vi "3-2 생산자소비자(이벤트).vi"() -> ()   [LabVIEW 2014]
uses:
  <vilib>/Analysis/NI_AALBase.lvlib
panel:
  in  "기다림":i32
  out "웨이브폼 그래프":dbl[](graph)
  in  "정지":bool
  in  "확인 버튼":bool
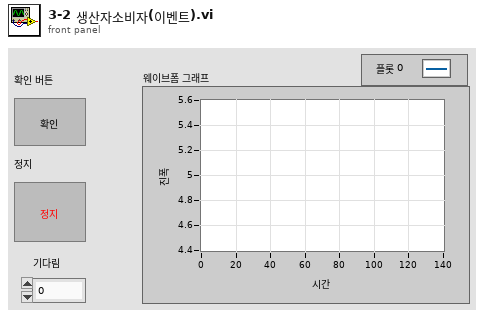
[diagram p1: front panel]
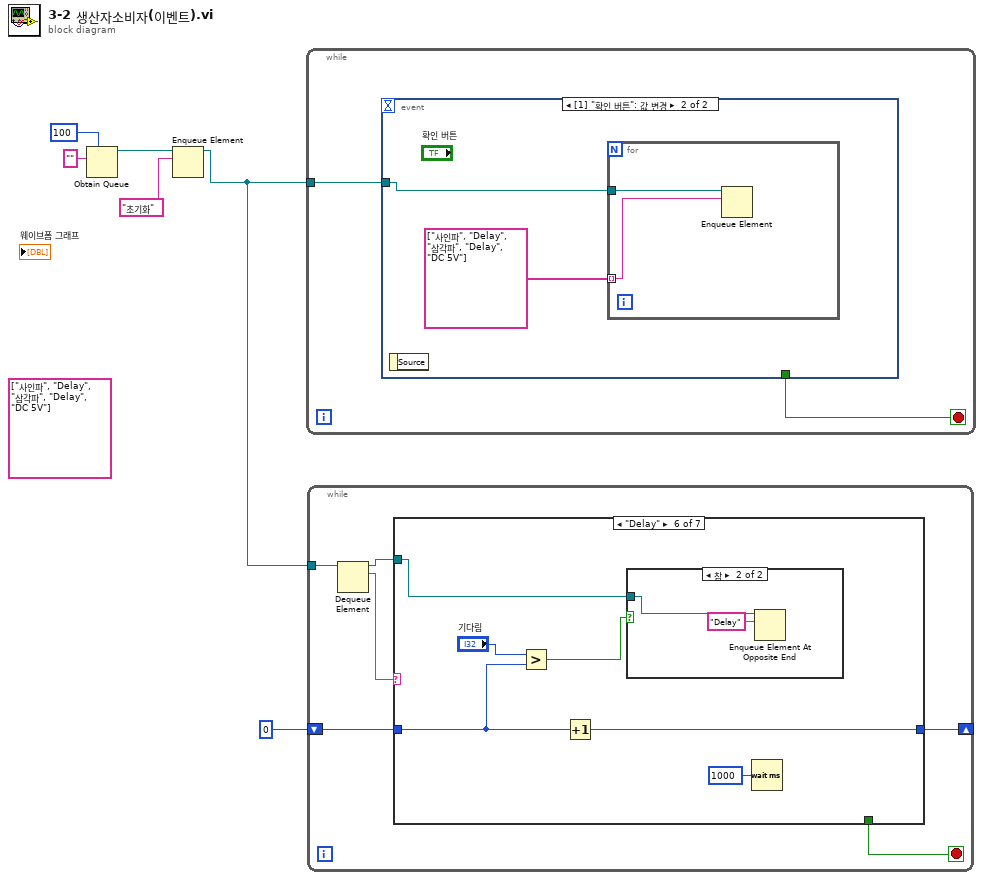
[diagram p0: block diagram]
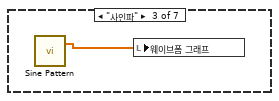
[diagram p4: hidden frame]
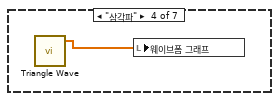
[diagram p5: hidden frame]
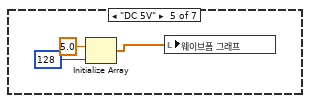
[diagram p6: hidden frame]
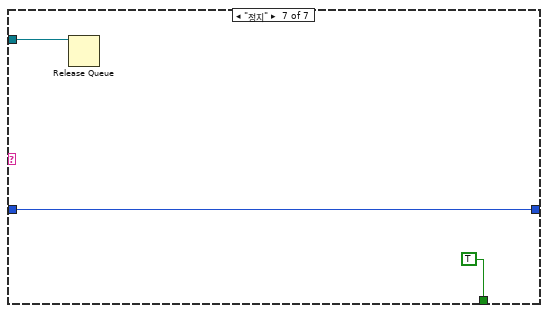
[diagram p8: hidden frame]
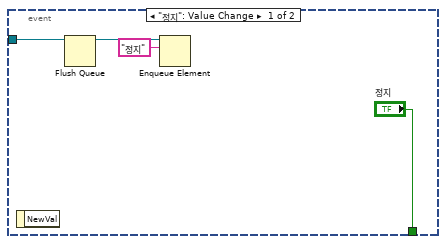
[diagram p9: hidden frame]
diagram:
  (unwired) string[] ["사인파", "Delay", "삼각파", "Delay", "DC 5V"]
  n1 = Obtain Queue(max queue size (-1, unlimited)=100 ("최대 큐 크기(-1,제한없음)"), element data type="" ("원소 데이터 타입")) -> (queue out=w4:refnum<queue>)  [unwired: 3 in, 2 out]
  n2 = Enqueue Element(queue=w4, element="초기화" ("원소")) -> (queue out=w3:refnum<queue>)  [unwired: 2 in, 2 out]
  n3 = while {
    tunnel: w3 -> [w7]
    stop <- w8 stop-if-true
    n4 = event shown="[1] \"확인 버튼\": 값 변경" {
      selector: _ -> [_ _]
      dyn-events: _ -> [_ _]
      timeout: _ -> [_ _]
      tunnel: ["정지" _] -> w8
      tunnel: w7 -> [w9 w14]
      event "정지": Value Change {
        n5 = event-data() -> ()  [unwired: 1 in, 1 out]
        n6 = Flush Queue(queue=w9) -> (queue out=w11:refnum<queue>)  [unwired: 1 in, 2 out]
        n7 = Enqueue Element(queue=w11, element="정지" ("원소")) -> ()  [unwired: 2 in, 3 out]
      }
      event "확인 버튼": Value Change {
        n8 = event-data() -> ()  [unwired: 1 in, 1 out]
        n9 = for {
          tunnel: w14 -> [w16]
          tunnel: string[] ["사인파", "Delay", "삼각파", "Delay", "DC 5V"] -> [w15] mode=indexing
          n10 = Enqueue Element(queue=w16, element=w15) -> ()  [unwired: 2 in, 3 out]
        }
      }
    }
  }
  n11 = while {
    tunnel: w3 -> [w22]
    shift-right: [w17] -> _
    shift-left: 0 -> [w18]
    stop <- w19 stop-if-true
    n12 = Dequeue Element(queue=w22) -> (queue out=w20:refnum<queue>, element=w21:string)  [unwired: 2 in, 2 out]
    n13 = case shown="\"Delay\"" w21 {
      tunnel: w20 -> [_ _ _ _ _ w33 w38]
      tunnel: [_ _ _ _ _ _ TRUE] -> w19
      tunnel: w18 -> [_ _ _ _ _ w30 w36]
      tunnel: [_ _ _ _ _ w32 w36] -> w17
      frame "기본", Default {
      }
      frame "초기화" {
      }
      frame "사인파" {
        n14 = call <vilib>:"Sine Pattern.vi"() -> ("Sinusoidal Pattern"=w23:dbl[])  [unwired: 4 in, 1 out]
        n15 = local write "웨이브폼 그래프"(w23) -> ()
      }
      frame "삼각파" {
        n16 = call <vilib>:"Triangle Wave.vi"() -> ("triangle wave"=w24:dbl[])  [unwired: 5 in, 2 out]
        n17 = local write "웨이브폼 그래프"(w24) -> ()
      }
      frame "DC 5V" {
        n18 = Initialize Array(5.0 ("원소"), 128 ("차원 크기")) -> (w25:dbl[])
        n19 = local write "웨이브폼 그래프"(w25) -> ()
      }
      frame "Delay" {
        n20 = Greater?(x="기다림", y=w30) -> (0:w28:bool)
        n21 = Increment(x=w30) -> (x+1=w32:i32)
        n22 = case shown="참" w28 {
          tunnel: w33 -> [_ w35]
          frame False {
          }
          frame True {
            n23 = Enqueue Element At Opposite End(queue=w35, element="Delay" ("원소")) -> ()  [unwired: 2 in, 3 out]
          }
        }
        n24 = Wait (ms)(milliseconds to wait=u32 1000 ("대기 시간(ms)")) -> ()  [unwired: 1 out]
      }
      frame "정지" {
        n25 = Release Queue(queue=w38) -> ()  [unwired: 2 in, 3 out]
      }
    }
  }
